vi "SLSC Convert Items - String to Variants.vi"(0 "Datatype":string, 5 "Value":string, 12 "enums":T1[](array[typedef])) -> (4 "Datatype found?":bool, 6 "enum":T1, 8 "Value":variant)   [LabVIEW 2017, in "SLSC Tree Control.lvlib"]
doc: "Converts the string values of the tree control to variants and doubles datatypes."
uses:
  SLSC Tree Control.lvlib
  Ctrl/Enum.ctl
  Ctrl/EnumValue.ctl
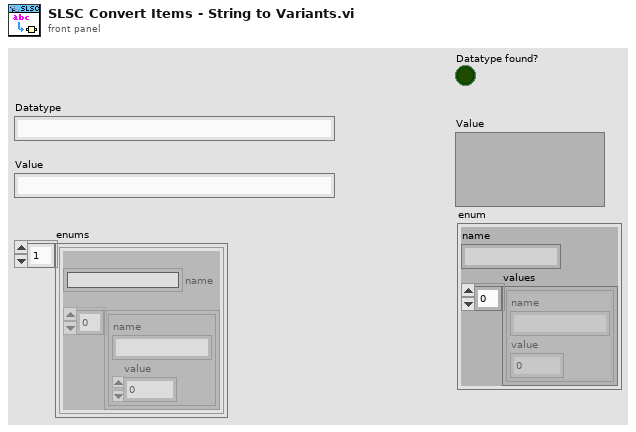
[diagram p1: front panel]
types:
  T1 = typedef "Enum.ctl" = cluster{"name":string, "values":T2[]}
  T2 = typedef "EnumValue.ctl" = cluster{"name":string, "value":i32}
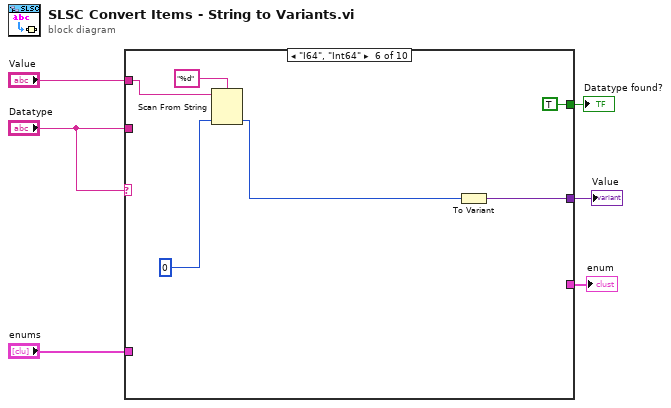
[diagram p0: block diagram]
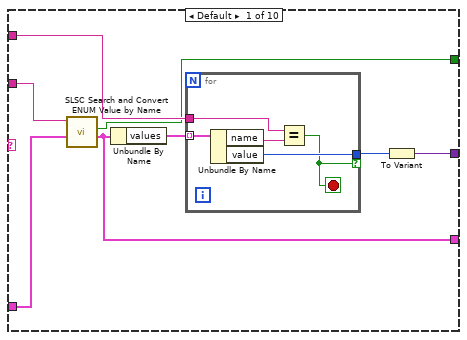
[diagram p2: hidden frame]
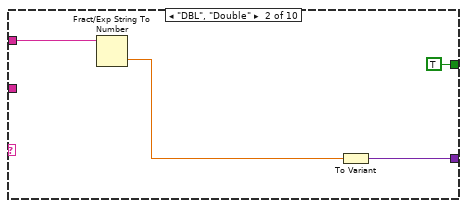
[diagram p3: hidden frame]
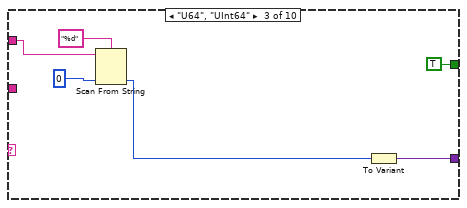
[diagram p4: hidden frame]
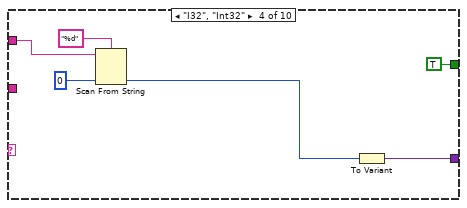
[diagram p5: hidden frame]
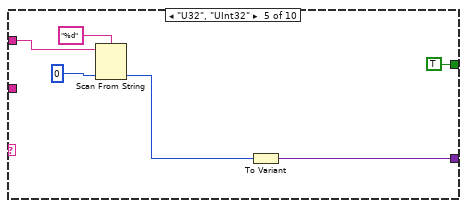
[diagram p6: hidden frame]
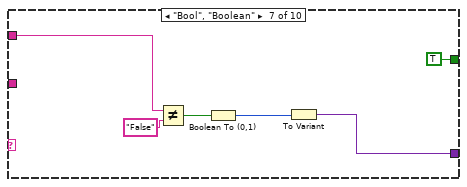
[diagram p7: hidden frame]
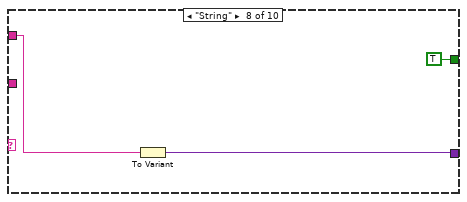
[diagram p8: hidden frame]
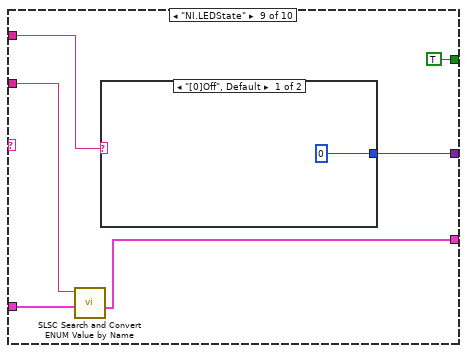
[diagram p9: hidden frame]
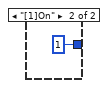
[diagram p10: hidden frame]
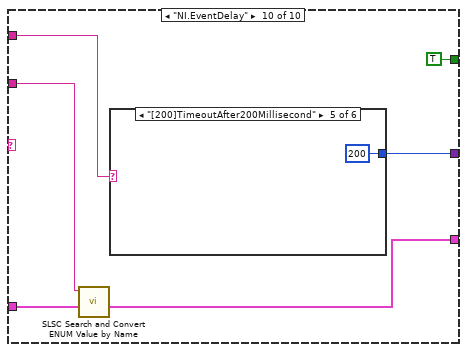
[diagram p11: hidden frame]
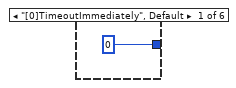
[diagram p12: hidden frame]
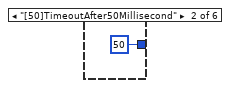
[diagram p13: hidden frame]
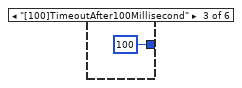
[diagram p14: hidden frame]
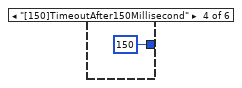
[diagram p15: hidden frame]
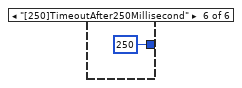
[diagram p16: hidden frame]
diagram:
  n1 = case shown="\"I64\", \"Int64\"" "Datatype" {
    tunnel: "Datatype" -> [w14 _ _ _ _ _ _ _ w59 w67]
    tunnel: "enums" -> [w13 _ _ _ _ _ _ _ w58 w66]
    tunnel: "Value" -> [w11 w23 w29 w33 w41 w47 w52 w56 w61 w69]
    tunnel: [w9 w21 w25 w31 w37 w43 w49 w55 w60 w68] -> w3
    tunnel: [w8 _ _ _ _ _ _ _ w57 w65] -> w2
    tunnel: [w7 TRUE ("Datatype found?") TRUE ("Datatype found?") TRUE ("Datatype found?") TRUE ("Datatype found?") TRUE ("Datatype found?") TRUE ("Datatype found?") TRUE ("Datatype found?") TRUE ("Datatype found?") TRUE ("Datatype found?")] -> w1
    frame Default {
      n2 = call "SLSC Search and Convert ENUM Value by Name.vi"("enums"=w13, "Datatype Name"=w14) -> ("Enum"=w8:T1, "Datatype found?"=w7:bool)  [unwired: 8 in]
      n3 = Unbundle By Name(w8) -> ("values"=w12:T2[])
      n4 = for {
        tunnel: w12 -> [w19] mode=indexing
        tunnel: w11 -> [w17]
        tunnel: [w16] -> w10 if=w15
        stop <- w15 stop-if-true
        n5 = Unbundle By Name(w19) -> ("name"=w18:string, "value"=w16:i32)
        n6 = Equal?(x=w17, y=w18) -> (x = y?=w15:bool)
      }
      n7 = To Variant(anything=w10) -> (Variant=w9:variant)
    }
    frame "DBL", "Double" {
      n8 = Fract/Exp String To Number(string=w23) -> (number=w22:dbl)  [unwired: 3 in, 1 out]
      n9 = To Variant(anything=w22) -> (Variant=w21:variant)
    }
    frame "U64", "UInt64" {
      n10 = Scan From String(format string="%d", input string=w29, default 1=u64 0 ("default (0 U32)")) -> (output 1=w26:u64)  [unwired: 2 in, 3 out]
      n11 = To Variant(anything=w26) -> (Variant=w25:variant)
    }
    frame "I32", "Int32" {
      n12 = Scan From String(format string="%d", input string=w33, default 1=0 ("default (0 U32)")) -> (output 1=w32:i32)  [unwired: 2 in, 3 out]
      n13 = To Variant(anything=w32) -> (Variant=w31:variant)
    }
    frame "U32", "UInt32" {
      n14 = Scan From String(format string="%d", input string=w41, default 1=u32 0 ("default (0 U32)")) -> (output 1=w38:u32)  [unwired: 2 in, 3 out]
      n15 = To Variant(anything=w38) -> (Variant=w37:variant)
    }
    frame "I64", "Int64" {
      n16 = Scan From String(format string="%d", input string=w47, default 1=i64 0 ("default (0 U32)")) -> (output 1=w44:i64)  [unwired: 2 in, 3 out]
      n17 = To Variant(anything=w44) -> (Variant=w43:variant)
    }
    frame "Bool", "Boolean" {
      n18 = Not Equal?(x=w52, y="False") -> (x != y?=w51:bool)
      n19 = Boolean To (0,1)(Boolean=w51) -> (0, 1=w50:i16)
      n20 = To Variant(anything=w50) -> (Variant=w49:variant)
    }
    frame "String" {
      n21 = To Variant(anything=w56) -> (Variant=w55:variant)
    }
    frame "NI.LEDState" {
      n22 = call "SLSC Search and Convert ENUM Value by Name.vi"("enums"=w58, "Datatype Name"=w59) -> ("Enum"=w57:T1)  [unwired: 8 in, 1 out]
      n23 = case shown="\"[0]Off\", Default" w61 {
        tunnel: [0 1] -> w60
        frame "[0]Off", Default {
        }
        frame "[1]On" {
        }
      }
    }
    frame "NI.EventDelay" {
      n24 = call "SLSC Search and Convert ENUM Value by Name.vi"("enums"=w66, "Datatype Name"=w67) -> ("Enum"=w65:T1)  [unwired: 8 in, 1 out]
      n25 = case shown="\"[200]TimeoutAfter200Millisecond\"" w69 {
        tunnel: [0 50 100 150 200 250] -> w68
        frame "[0]TimeoutImmediately", Default {
        }
        frame "[50]TimeoutAfter50Millisecond" {
        }
        frame "[100]TimeoutAfter100Millisecond" {
        }
        frame "[150]TimeoutAfter150Millisecond" {
        }
        frame "[200]TimeoutAfter200Millisecond" {
        }
        frame "[250]TimeoutAfter250Millisecond" {
        }
      }
    }
  }
  "Value" <- w3
  "enum" <- w2
  "Datatype found?" <- w1
